vi "AutoDrive.vi"(9 "Steady Val":dbl, 11 "Distance to travel (inches)":dbl) -> ()   [LabVIEW 2012]
uses:
  State_Machine_Enum.ctl
  Robot Global Data.vi
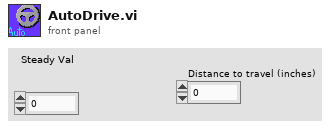
[diagram p1: front panel]
types:
  T1 = typedef "State_Machine_Enum.ctl" = enum16{"Idle", "Start", "Do", "Stop", "Init"}
  T2 = typedef "WPI_EncoderDevRef.ctl" = cluster{"DevStatus":errorcluster, "EncoderIndex":T3, "CounterIndex":T4, "DistancePerCount":dbl, "Decoding Type":T5}
  T3 = typedef "FPGA_EncoderIdx.ctl" = enum8{"Enc 0", "Enc 1", "Enc 2", "Enc 3", "Invalid"}
  T4 = typedef "FPGA_CounterCtrSystemIndex.ctl" = enum8{"Ctr 0", "Ctr 1", "Ctr 2", "Ctr 3", "Ctr 4", "Ctr 5", "Ctr 6", "Ctr 7", "Invalid"}
  T5 = typedef "WPI_EncoderType.ctl" = enum16{"1x", "2x", "4x"}
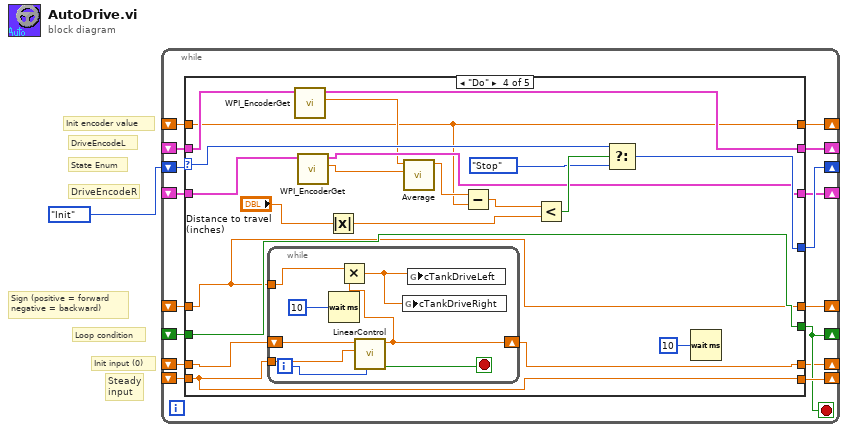
[diagram p0: block diagram]
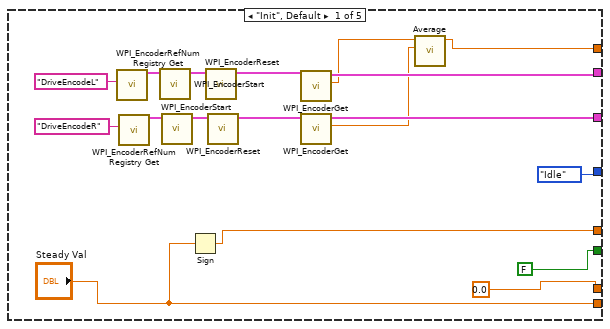
[diagram p2: hidden frame]
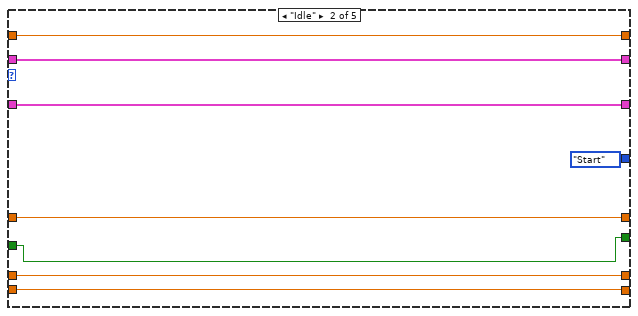
[diagram p3: hidden frame]
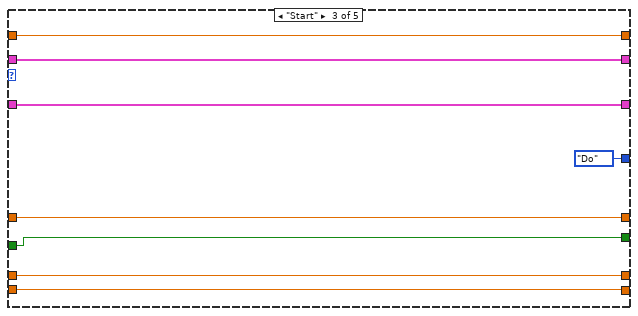
[diagram p4: hidden frame]
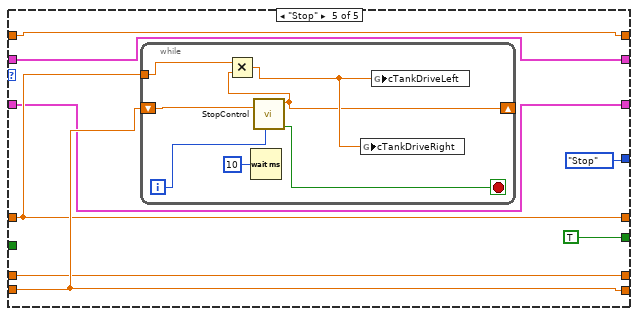
[diagram p5: hidden frame]
diagram:
  # "DriveEncodeR"
  # "DriveEncodeL"
  # "Sign (positive = forward\nnegative = backward)"
  # "Init encoder value"
  # "State Enum"
  # "Loop condition"
  # "Init input (0)"
  # "Steady\ninput"
  n1 = while {
    shift-right: [w16] -> _
    shift-left: State_Machine_Enum."Init" ("State") -> [w17]
    shift-right: [w15] -> _
    shift-left: _ -> [w14]
    shift-right: [w13] -> _
    shift-left: _ -> [w12]
    shift-right: [w11] -> _
    shift-left: _ -> [w10]
    shift-right: [w9] -> _
    shift-left: _ -> [w8]
    shift-right: [w7] -> _
    shift-left: _ -> [w6]
    shift-right: [w5] -> _
    shift-left: _ -> [w3]
    shift-right: [w4] -> _
    shift-left: _ -> [w2]
    stop <- w13 stop-if-true
    n2 = case shown="\"Do\"" w17 {
      selector: w17 -> [_ _ _ w72 _]
      tunnel: [State_Machine_Enum."Idle" ("State") State_Machine_Enum."Start" ("State") State_Machine_Enum."Do" ("State") w71 State_Machine_Enum."Stop" ("State")] -> w16
      tunnel: ["Steady Val" w43 w51 w68 w88] -> w15
      tunnel: w14 -> [_ w43 w51 w68 w88]
      tunnel: [FALSE w42 w50 w66 TRUE] -> w13
      tunnel: w12 -> [_ w42 w50 w66 _]
      tunnel: [0.0 ("New Motor Input") w41 w49 w64 w86] -> w11
      tunnel: w10 -> [_ w41 w49 w65 w86]
      tunnel: [w18 w40 w48 w52 w85] -> w9
      tunnel: w8 -> [_ w40 w48 w52 w85]
      tunnel: [w31 w38 w46 w60 w83] -> w7
      tunnel: w6 -> [_ w38 w46 w60 w83]
      tunnel: [w21 w37 w45 w57 w82] -> w5
      tunnel: [w23 w36 w44 w56 w81] -> w4
      tunnel: w3 -> [_ w37 w45 w59 w82]
      tunnel: w2 -> [_ w36 w44 w58 w81]
      frame "Init", Default {
        n3 = call <vilib>:"WPI_EncoderRefNum Registry Get.vi"("refnum name"="DriveEncodeL") -> ("EncoderDevRef"=w30:T2)  [unwired: 9 in, 1 out]
        n4 = call <vilib>:"WPI_EncoderRefNum Registry Get.vi"("refnum name"="DriveEncodeR") -> ("EncoderDevRef"=w27:T2)  [unwired: 9 in, 1 out]
        n5 = call <vilib>:"WPI_EncoderStart.vi"("EncoderDevRef"=w30) -> ("EncoderDevRef"=w28:T2)  [unwired: 1 in, 9 out]
        n6 = call <vilib>:"WPI_EncoderStart.vi"("EncoderDevRef"=w27) -> ("EncoderDevRef"=w25:T2)  [unwired: 1 in, 9 out]
        n7 = Sign(1:"Steady Val") -> (0:w31:dbl)
        n8 = call <vilib>:"WPI_EncoderReset.vi"("EncoderDevRef"=w28) -> ("EncoderDevRef"=w22:T2)  [unwired: 1 in, 9 out]
        n9 = call <vilib>:"WPI_EncoderReset.vi"("EncoderDevRef"=w25) -> ("EncoderDevRef"=w24:T2)  [unwired: 1 in, 9 out]
        n10 = call <vilib>:"WPI_EncoderGet.vi"("EncoderDevRef"=w22) -> ("Distance"=w20:dbl, "EncoderDevRef"=w21:T2)  [unwired: 5 in, 4 out]
        n11 = call <vilib>:"WPI_EncoderGet.vi"("EncoderDevRef"=w24) -> ("Distance"=w19:dbl, "EncoderDevRef"=w23:T2)  [unwired: 5 in, 4 out]
        n12 = call "Average.vi"("y"=w19, "x"=w20) -> ("x/y"=w18:dbl)  [unwired: 9 in]
      }
      frame "Idle" {
      }
      frame "Start" {
      }
      frame "Do" {
        n13 = while {
          shift-right: [w74] -> w64
          shift-left: w65 -> [w80]
          tunnel: w68 -> [w79]
          tunnel: w60 -> [w77]
          i -> [w73]
          stop <- w75 stop-if-true
          n14 = Wait (ms)(milliseconds to wait=u32 10) -> ()  [unwired: 1 out]
          n15 = call "LinearControl.vi"("Loop Iteration"=w73, "Setpoint"=w79, "Motor Value"=w80) -> ("Currently Matching"=w75:bool, "New Motor Value"=w74:dbl)  [unwired: 7 in]
          n16 = Multiply(x=w77, y=w74) -> (x*y=w76:dbl)
          n17 = global write "Robot Global Data.vi" "cTankDriveRight"(w76) -> ()
          n18 = global write "Robot Global Data.vi" "cTankDriveLeft"(w76) -> ()
        }
        n19 = call <vilib>:"WPI_EncoderGet.vi"("EncoderDevRef"=w59) -> ("Distance"=w55:dbl, "EncoderDevRef"=w57:T2)  [unwired: 5 in, 4 out]
        n20 = call <vilib>:"WPI_EncoderGet.vi"("EncoderDevRef"=w58) -> ("Distance"=w54:dbl, "EncoderDevRef"=w56:T2)  [unwired: 5 in, 4 out]
        n21 = Absolute Value(x="Distance to travel (inches)") -> (abs(x)=w61:dbl)
        n22 = call "Average.vi"("y"=w54, "x"=w55) -> ("x/y"=w53:dbl)  [unwired: 9 in]
        n23 = Subtract(x=w53, y=w52) -> (x-y=w63:dbl)
        n24 = Less?(x=w63, y=w61) -> (x < y?=w69:bool)
        n25 = Select(t=w72, s=w69, f=State_Machine_Enum."Stop" ("State")) -> (s? t:f=w71:T1)
        n26 = Wait (ms)(milliseconds to wait=u32 10) -> ()  [unwired: 1 out]
      }
      frame "Stop" {
        n27 = while {
          shift-right: [w92] -> _
          shift-left: w88 -> [w95]
          tunnel: w83 -> [w94]
          i -> [w89]
          stop <- w91 stop-if-true
          n28 = Wait (ms)(milliseconds to wait=u32 10) -> ()  [unwired: 1 out]
          n29 = call "StopControl.vi"("Loop Iteration"=w89, "Motor Value"=w95) -> ("Done Stopping"=w91:bool, "New Motor Value"=w92:dbl)  [unwired: 8 in]
          n30 = Multiply(x=w94, y=w92) -> (x*y=w93:dbl)
          n31 = global write "Robot Global Data.vi" "cTankDriveRight"(w93) -> ()
          n32 = global write "Robot Global Data.vi" "cTankDriveLeft"(w93) -> ()
        }
      }
    }
  }
